vi "Memory.Pointer.Read Bytes.Subset.In Place.vi"   [LabVIEW 2016, in "LabVIEW Memory Manager.lvlib" / "Memory.Pointer.lvclass"]
uses:
  Memory.Pointer.lvclass
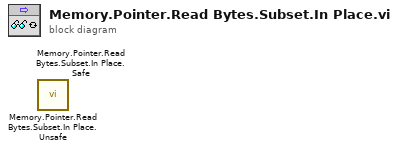
[diagram p0: block diagram]
diagram:
  n1 = call "Memory.Pointer.Read Bytes.Subset.In Place.Unsafe.vi"() -> ()  [unwired: 8 in, 4 out]
  n2 = call "Memory.Pointer.Read Bytes.Subset.In Place.Safe.vi"() -> ()  [unwired: 8 in, 4 out]
